vi "PID control.vi"(6 "reinitialize? (F)":bool, 8 "error in":errorcluster) -> (0 "error out":errorcluster, 3 "output":dbl)   [LabVIEW 2018]
uses:
  <vilib>/addons/control/pid/pid.llb/PID (DBL).vi
  <vilib>/addons/control/pid/NI_PID_pid.lvlib
panel:
  in  "setpoint":dbl(slide) scale=0.0..10.0
  out "Servo Angle":i16
  out "X_Pos":dbl
  in  "output range":cluster{"output high":dbl, "output low":dbl}={"output high"=50.0, "output low"=-50.0} {"output low" format="%.2f"; "output high" format="%.2f"}
  in  "dt (s)":dbl=-1.0 format="%.3f"
  in  "PID gains":T1={"proportional gain (Kc)"=1.0, "integral time (Ti, min)"=0.01, "derivative time (Td, min)"=0.0} {"derivative time (Td, min)" format="%.3f"; "integral time (Ti, min)" format="%.3f"; "proportional gain (Kc)" format="%.3f"}
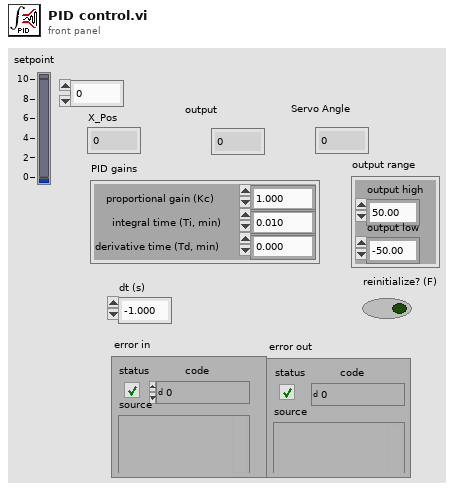
[diagram p1: front panel]
types:
  T1 = cluster{"proportional gain (Kc)":dbl, "integral time (Ti, min)":dbl, "derivative time (Td, min)":dbl}
  T2 = cluster{"Pos. X":i32, "Pos. Y":i32, "Radius":i32, "Core Area":i32}
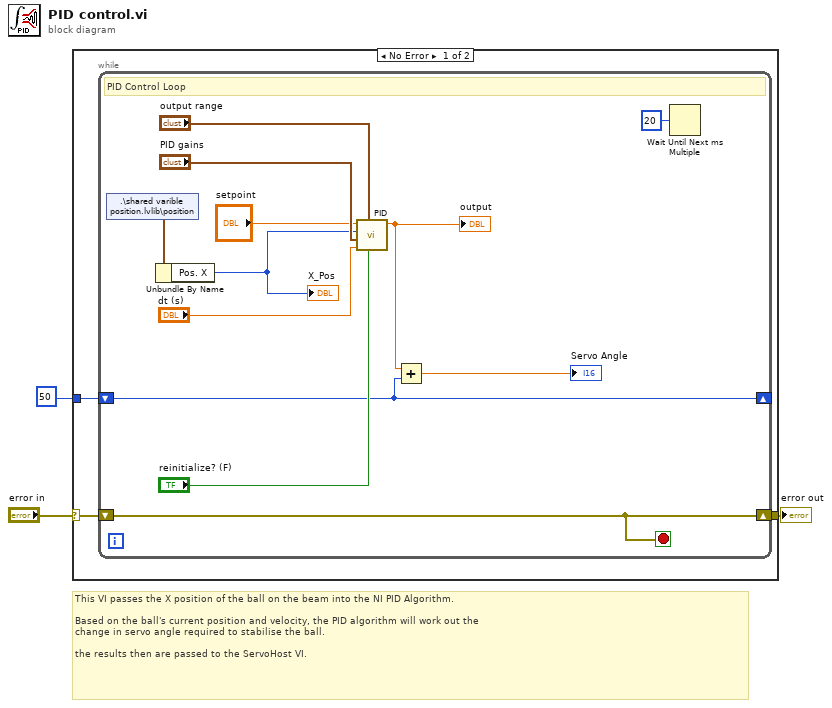
[diagram p0: block diagram]
diagram:
  # "This VI passes the X position of the ball on the beam into the NI PID Algorithm.\n\nBased on the ball's current position and velocity, the PID algorithm will work out the\nchange in servo angle required to stabilise the ball. \n\nthe results then are passed to the ServoHost VI."
  n1 = case shown="No Error" "error in" {
    selector: "error in" -> [w6 w19]
    tunnel: [w5 w19] -> w2
    tunnel: 50 -> [w4 _]
    frame No Error {
      n2 = while {
        shift-right: [w11] -> _
        shift-left: w4 -> [w11]
        shift-right: [w13] -> w5
        shift-left: w6 -> [w13]
        stop <- w13 stop-if-true
        # "PID Control Loop"
        n3 = shared-variable ".\\shared varible position.lvlib\\position"() -> (w9:T2)  [unwired: 1 in, 1 out]
        n4 = Unbundle By Name(w9) -> ("Pos. X"=w8:i32)
        "X_Pos" <- w8
        n5 = call-poly <vilib>:"PID.vi"("reinitialize? (F)"="reinitialize? (F)", "output range"="output range", "dt (s)"="dt (s)", "PID gains"="PID gains", "process variable"=w8, "setpoint"="setpoint") -> ("output"=w12:dbl)  [unwired: 4 in, 1 out]
        "output" <- w12
        n6 = Add(x=w12, y=w11) -> (x+y=→"Servo Angle":dbl)
        n7 = Wait Until Next ms Multiple(millisecond multiple=u32 20) -> ()  [unwired: 1 out]
      }
    }
    frame Error {
      # "Do nothing in error case"
    }
  }
  "error out" <- w2
